vi "add_and_configure_target.vi"(8 "error in":errorcluster, 10 "Target Configuration":T1, 11 "vsd reference":refnum<k24>) -> (0 "error out":errorcluster, 2 "target ref":refnum<k24>, 3 "vsd reference out":refnum<k24>)   [LabVIEW 2020]
uses:
  NationalInstruments.VeriStand.SystemDefinitionAPI
  controls/target_configuration_cluster.ctl
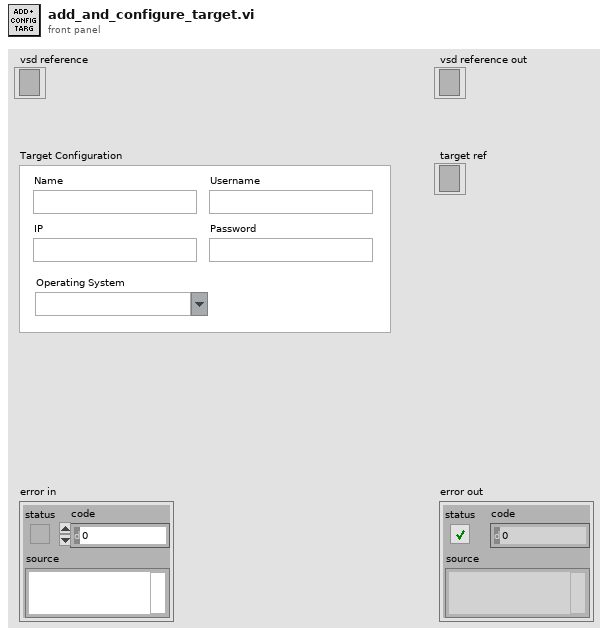
[diagram p1: front panel]
types:
  T1 = typedef "target_configuration_cluster.ctl" = cluster{"Name":string, "IP":string, "Username":string, "Password":string, "Operating System":string}
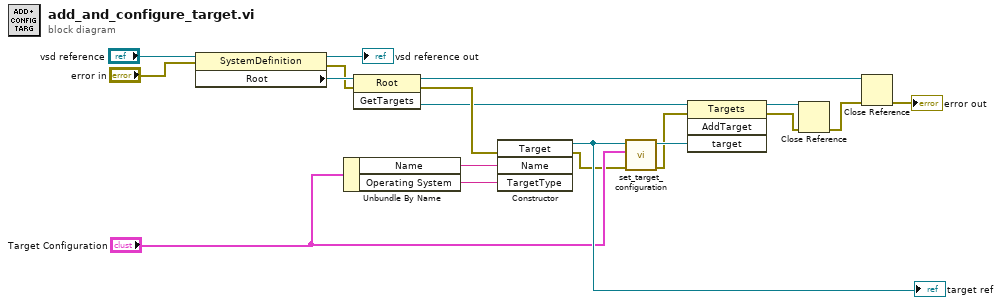
[diagram p0: block diagram]
diagram:
  n1 = property class="SystemDefinition"(reference="vsd reference", error in="error in") -> (reference out=→"vsd reference out":refnum<k24>, error out=w16:errorcluster, "Root"=w19:refnum<k24>)
  n2 = Unbundle By Name("Target Configuration") -> ("Name"=w7:string, "Operating System"=w6:string)
  n3 = invoke class="Root" method="GetTargets"(reference=w19, error in=w16) -> (reference out=w14:refnum<k24>, error out=w17:errorcluster, "GetTargets"=w8:refnum<k24>)  [unwired: 1 in]
  n4 = constructor class="Target"(error in=w17, "Name"=w7, "TargetType"=w6) -> (reference out=w5:refnum<k24>, error out=w1:errorcluster)  [unwired: 2 in, 3 out]
  "target ref" <- w5
  n5 = call "set_target_configuration.vi"("error in"=w1, "Target Configuration Data"="Target Configuration", "target ref"=w5) -> ("error out"=w2:errorcluster, "target ref out"=w4:refnum<k24>)  [unwired: 7 in]
  n6 = invoke class="Targets" method="AddTarget"(reference=w8, error in=w2, "target"=w4) -> (reference out=w12:refnum<k24>, error out=w11:errorcluster)  [unwired: 1 in, 2 out]
  n7 = Close Reference(reference=w12, error in (no error)=w11) -> (error out=w10:errorcluster)
  n8 = Close Reference(reference=w14, error in (no error)=w10) -> (error out=→"error out":errorcluster)
